vi "Configure Pressure.vi"(0 "VISA resource name":refnum<visa-resource-name>, 1 "Low RPT Pressure Offset (0)":dbl, 5 "BPR Mode (2: Auto)":u16(ring)=2 items=["Off", "On", "Auto"], 7 "Enable BPR Suspension (Enable)":bool=TRUE, 9 "High RPT Pressure Offset (0)":dbl, 11 "error in (no error)":errorcluster, 12 "Internal Pressure Transducer Upper Limit (500 kPa)":dbl=500.0) -> (4 "VISA resource name out":refnum<visa-resource-name>, 15 "error out":errorcluster)   [LabVIEW 2023, in "Fluke Molbox 1 Plus.lvlib"]
doc: "Configures pressure for the instrument including BPR (back pressure ratio), internal pressure transducer, and RPT pressure."
uses:
  Fluke Molbox 1 Plus.lvlib
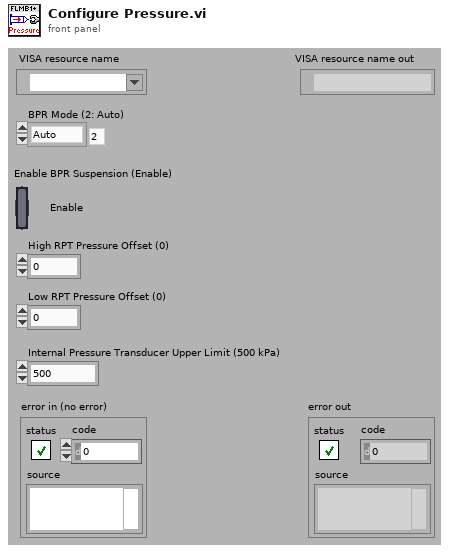
[diagram p1: front panel]
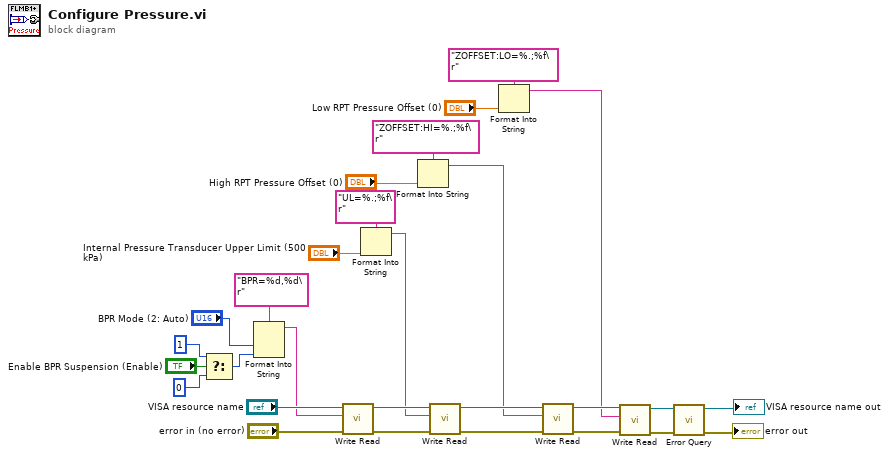
[diagram p0: block diagram]
diagram:
  n1 = Select(t=1, s="Enable BPR Suspension (Enable)", f=0) -> (s? t:f=w24:i32)
  n2 = Format Into String(format string="BPR=%d,%d\r", "BPR Mode (2: Auto)", w24) -> (resulting string=w14:string)  [unwired: 2 in, 1 out]
  n3 = call "Write Read.vi"("error in (no error)"="error in (no error)", "Write String"=w14, "VISA resource name"="VISA resource name") -> ("error out"=w12:errorcluster, "VISA resource name out"=w13:refnum<visa-resource-name>)  [unwired: 6 in, 1 out]
  n4 = Format Into String(format string="UL=%.;%f\r", "Internal Pressure Transducer Upper Limit (500 kPa)") -> (resulting string=w11:string)  [unwired: 2 in, 1 out]
  n5 = Format Into String(format string="ZOFFSET:HI=%.;%f\r", "High RPT Pressure Offset (0)") -> (resulting string=w9:string)  [unwired: 2 in, 1 out]
  n6 = call "Write Read.vi"("error in (no error)"=w12, "Write String"=w11, "VISA resource name"=w13) -> ("error out"=w8:errorcluster, "VISA resource name out"=w10:refnum<visa-resource-name>)  [unwired: 6 in, 1 out]
  n7 = Format Into String(format string="ZOFFSET:LO=%.;%f\r", "Low RPT Pressure Offset (0)") -> (resulting string=w5:string)  [unwired: 2 in, 1 out]
  n8 = call "Write Read.vi"("error in (no error)"=w8, "Write String"=w9, "VISA resource name"=w10) -> ("error out"=w6:errorcluster, "VISA resource name out"=w7:refnum<visa-resource-name>)  [unwired: 6 in, 1 out]
  n9 = call "Write Read.vi"("error in (no error)"=w6, "Write String"=w5, "VISA resource name"=w7) -> ("error out"=w3:errorcluster, "VISA resource name out"=w4:refnum<visa-resource-name>)  [unwired: 6 in, 1 out]
  n10 = call "Error Query.vi"("error in (no error)"=w3, "VISA resource name"=w4) -> ("error out"=→"error out":errorcluster, "VISA resource name out"=→"VISA resource name out":refnum<visa-resource-name>)  [unwired: 6 in, 2 out]
